vi "Handle Last Ack Core.vi"(4 "error in (no error)":errorcluster, 6 "Last Ack":refnum<class "Last Ack.lvclass">, 7 "IMAQ Display in":refnum<class "HIJ Vision Display.lvclass">) -> (0 "error out":errorcluster, 3 "IMAQ Display out":refnum<class "HIJ Vision Display.lvclass">)   [LabVIEW 2014, in "HIJ Vision Display.lvlib" / "HIJ Vision Display.lvclass"]
doc: "(<B>Filename</B>: Actor Framework.lvlib:Actor.lvclass:Handle Last Ack Core.vi)\n\nDefines how the caller actor responds to the Last Ack message from a nested actor. The Last Ack message is the final message a nested actor sends to its caller before it shuts down. The message contains information about the final state of the nested actor.\n\nBy default, this method does nothing except return any error the nested actor sent. A descendant class may override this method to define behavior."
uses:
  HIJ Vision Display.lvclass
  <vilib>/ActorFramework/LastAck/Last Ack.lvclass
  Select Report File Dialog/Select Report File Dialog/Select Report File Dialog.lvclass
  ROI Name Dialog/Select Report File Dialog/ROI Name Dialog.lvclass
  <vilib>/ActorFramework/LastAck/Last Ack.lvclass/Last Ack.ctl
  <vilib>/ActorFramework/Actor/Actor.lvclass/Actor.ctl
  <vilib>/ActorFramework/Message Enqueuer/Message Enqueuer.lvclass/Message Enqueuer.ctl
  Select Report File Dialog/Select Report File Dialog/Select Report File Dialog.lvclass/Select Report File Dialog.ctl
  HIJ Vision Display Messages/Load ROI from File Msg/Load ROI from File Msg.lvclass/Load ROI from File Msg.ctl
  ROI Name Dialog/Select Report File Dialog/ROI Name Dialog.lvclass/ROI Name Dialog.ctl
  HIJ Vision Display.lvclass/HIJ Vision Display.ctl
  <vilib>/ActorFramework/Message Enqueuer/Init from Existing Queue.vi
  <vilib>/ActorFramework/Message Enqueuer/Enqueue.vi
  <vilib>/ActorFramework/Message Priority Queue/Priority Enqueue.vi
  Shared Code/Viewable Actor/ViewableActor/ViewableActor.lvclass
  <vilib>/ActorFramework/Message Enqueuer/Message Enqueuer.lvclass
  HIJ Vision Display Messages/Load ROI from File Msg/Load ROI from File Msg.lvclass
  <vilib>/ActorFramework/Actor/Actor.lvclass
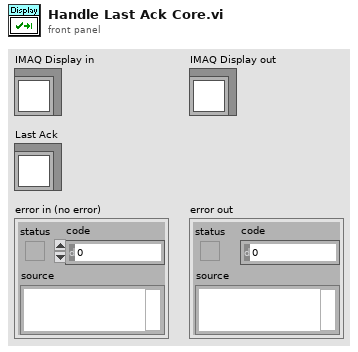
[diagram p1: front panel]
types:
  T1 = typedef "HIJ Vision Display.lvlib/HIJ Vision Display.lvclass/Named ROI.ctl" = cluster{"ROI":cluster{"Global Rectangle":i32[], "Contours":cluster{"Contour Type":u32, "ROI Type":u32, "Points":i32[]}[]}, "Name":string}
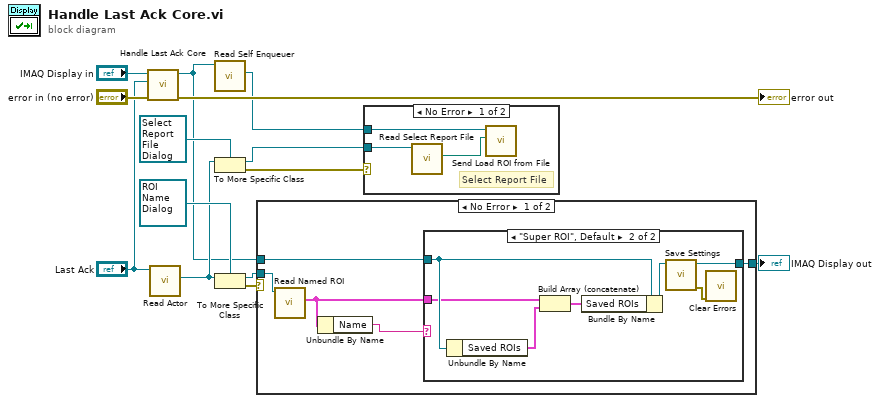
[diagram p0: block diagram]
diagram:
  n1 = call-parent "Handle Last Ack Core.vi"("error in (no error)"="error in (no error)", "Last Ack"="Last Ack", "Actor in"="IMAQ Display in") -> ("error out"=→"error out":errorcluster, "Actor out"=w2:refnum<class "HIJ Vision Display.lvclass">)  [unwired: 3 in]
  n2 = call <vilib>:"Read Actor.vi"("Last Ack"="Last Ack") -> ("Actor"=w5:refnum<class "Actor.lvclass">)  [unwired: 10 in]
  n3 = call <vilib>:"Read Self Enqueuer.vi"("Actor"=w2) -> ("Self Enqueuer"=w7:refnum<class "Message Enqueuer.lvclass">)  [unwired: 10 in]
  n4 = To More Specific Class(target class=refnum<class "Select Report File Dialog.lvclass"> refnum ("Select Report File Dialog.lvlib:Select Report File Dialog.lvclass"), reference=w5) -> (specific class reference=w8:refnum<class "Select Report File Dialog.lvclass">, error out=w9:errorcluster)  [unwired: 1 in]
  n5 = To More Specific Class(target class=refnum<class "ROI Name Dialog.lvclass"> refnum ("ROI Name Dialog.lvlib:ROI Name Dialog.lvclass"), reference=w5) -> (specific class reference=w4:refnum<class "ROI Name Dialog.lvclass">, error out=w3:errorcluster)  [unwired: 1 in]
  n6 = case shown="No Error" w3 {
    tunnel: w4 -> [w19 _]
    tunnel: w2 -> [w18 w28]
    tunnel: [w17 w28] -> w1
    frame No Error {
      n7 = call "Read Named ROI.vi"("ROI Name Dialog in"=w19) -> ("Named ROI"=w16:T1)  [unwired: 8 in, 2 out]
      n8 = Unbundle By Name(w16) -> ("Name"=w15:string)
      n9 = case shown="\"Super ROI\", Default" w15 {
        tunnel: w18 -> [w20 w25]
        tunnel: w16 -> [_ w24]
        tunnel: [w20 w22] -> w17
        frame "" {
        }
        frame "Super ROI", Default {
          n10 = Unbundle By Name(w25) -> ("Saved ROIs"=w26:T1[])
          n11 = Build Array (concatenate)(w24, w26) -> (w27:T1[])
          n12 = Bundle By Name(cluster=w25, "Saved ROIs"=w27) -> (w23:refnum<class "HIJ Vision Display.lvclass">)
          n13 = call-dynamic "Save Settings.vi"("IMAQ Display in"=w23) -> ("error out"=w21:errorcluster, "IMAQ Display out"=w22:refnum<class "HIJ Vision Display.lvclass">)  [unwired: 9 in]
          n14 = call <vilib>:"Clear Errors.vi"("error in (no error)"=w21) -> ()  [unwired: 5 in, 2 out]
        }
      }
    }
    frame Error {
    }
  }
  "IMAQ Display out" <- w1
  n15 = case shown="No Error" w9 {
    tunnel: w8 -> [w31 _]
    tunnel: w7 -> [w30 _]
    frame No Error {
      # "Select Report File"
      n16 = call "Read Select Report File.vi"("Select Report File Dialog in"=w31) -> ("Select Report File"=w29:path)  [unwired: 8 in, 2 out]
      n17 = call "Send Load ROI from File.vi"("Report File"=w29, "Message Enqueuer"=w30) -> ()  [unwired: 8 in, 2 out]
    }
    frame Error {
    }
  }
